vi "GetCurrentXYZPosition (SubVI).vi"(6 ".NET Refnum in - Device":refnum<k24>, 7 "error in (no error)":errorcluster, 10 "Axes Names":string[](array[string])) -> (0 "error out":errorcluster, 1 "Z Position Feedback":dbl, 2 "Y Position Feedback":dbl, 3 "X Position Feedback":dbl, 4 ".NET Refnum out  - Device":refnum<k24>)   [LabVIEW 2016]
uses:
  C:/Users/Aerotech/Documents/BNLStaveAssembly-blueprint/Bin/Aerotech.A3200.dll
  Bin/Aerotech.A3200.dll
panel:
  # "SubVI to retrieve the current position of the XYZ stage"
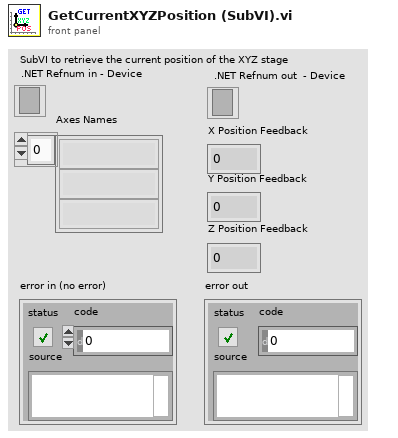
[diagram p1: front panel]
types:
  T1 = cluster{"Axes Names[0]":string, "Axes Names[1]":string, "Axes Names[2]":string, "Axes Names[3]":string, "Axes Names[4]":string, "Axes Names[5]":string, "Axes Names[6]":string, "Axes Names[7]":string, "Axes Names[8]":string}
  T2 = typedef "ControllerDiagPacket.ctl" = cluster{"Number of Diag Packets":i32, "Axes":T3[], "error":errorcluster}
  T3 = typedef "AxisDiagPacket.ctl" = cluster{"Axis Name":string, "Analog Input 0":dbl, "Analog Input 1":dbl, "Axis Fault (num)":i32, "Axis Fault (str)":string, "Axis Fault (bits)":cluster{"AmplifierFault":bool, "AmplifierTemperatureFault":bool, "CcwEndOfTravelLimitFault":bool, "CcwSoftwareLimitFault":bool, "CommunicationLostFault":bool, "CwEndOfTravelLimitFault":bool, "CwSoftwareLimitFault":bool, "EmergencyStopFault":bool, "EncoderFault":bool, "ExternalFault":bool, "FeedbackScalingFault":bool, "GantryMisalignFault ":bool, "HallSensorFault":bool, "InPositionTimeoutFault":bool, "MarkerSearchFault":bool, "MaxVelocityCommandFault":bool, "MissedInterruptFault":bool, "MotorTemperatureFault":bool, "None":bool, "OverCurrentFault":bool, "PositionErrorFault":bool, "PositionFeedbackFault":bool, "PowerSupplyFault":bool, "ProbeInputFault":bool, "SafeZoneFault":bool, "VelocityErrorFault":bool, "VelocityFeedbackFault":bool, "VoltageClampFault":bool}, "Axis Status (num)":i32, "Axis Status (str)":string, "Axis Status (bits)":cluster{"BacklashActive":bool, "CalibrationEnabled1D":bool, "CalibrationEnabled2D":bool, "CommandValid":bool, "DriveAbortPending":bool, "DrivePending":bool, "Enabling":bool, "GainMappingEnabled":bool, "GantryAligned":bool, "GantryRealigning":bool, "Homed":bool, "Homing":bool, "IFOVEnabled":bool, "JogGenerating":bool, "Jogging":bool, "JoystickControl":bool, "MasterSlaveControl":bool, "MotionBlocked":bool, "MotionClamped":bool, "MoveDone":bool, "None":bool, "NotVirtual":bool, "Profiling":bool, "Stability0":bool, "Stability1":bool, "TrajectoryFiltering":bool, "WaitDone":bool}, "Current Command":sgl, "Current Error":sgl, "Current Feedback":sgl, "Digital Inputs":i32, "Digital Outputs":i32, "Drive Status":i32, "Drive Status (str)":string, "Drive Status (bits)":cluster{"AccelerationPhase":bool, "AutofocusActive":bool, "BrakeOutput":bool, "CcwEndOfTravelLimitInput":bool, "CosineEncoderError":bool, "CurrentClamp":bool, "CwEndOfTravelLimitInput":bool, "DecelerationPhase":bool, "DualLoopActive":bool, "EmergencyStopInput":bool, "Enabled":bool, "EncoderClipping":bool, "GalvoCalibrationEnabled":bool, "GalvoPowerCorrection":bool, "HallAInput":bool, "HallBInput":bool, "HallCInput":bool, "HighResolutionMode":bool, "HomeLimitInput":bool, "InPosition":bool, "InPosition2":bool, "MarkerInput":bool, "MarkerLatch":bool, "MoveActive":bool, "NoMotorSupply":bool, "None":bool, "PowerLimiting":bool, "ProgrammingFlash":bool, "ProgrammingMXH":bool, "PSOHaltLatch":bool, "ServoControl":bool, "SineEncoderError":bool}, "Position Feedback Auxiliary":dbl, "Position Command":dbl, "Position Error":dbl, "Position Feedback":dbl, "Program Position Command":dbl, "Program Position Error":dbl, "Program Position Feedback":dbl, "Velocity Command":dbl, "Velocity Error":dbl, "Velocity Feedback":dbl}
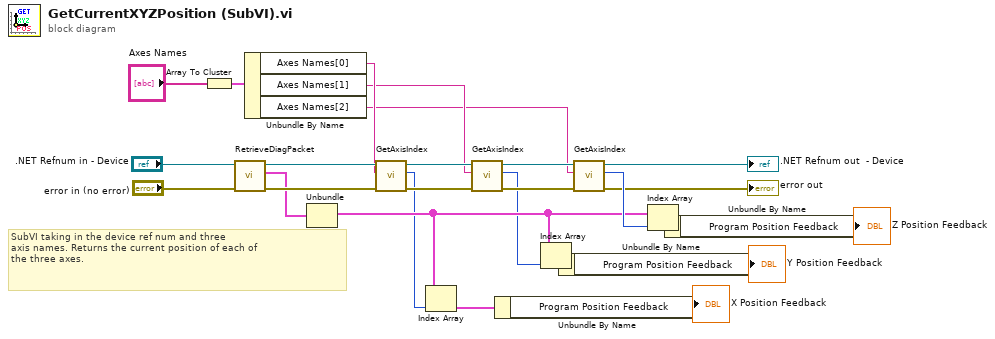
[diagram p0: block diagram]
diagram:
  # "SubVI taking in the device ref num and three\naxis names. Returns the current position of each of\nthe three axes."
  n1 = Array To Cluster(array="Axes Names") -> (cluster=w4:T1)
  n2 = call "RetrieveDiagPacket.vi"("error in (no error)"="error in (no error)", "Controller In"=".NET Refnum in - Device") -> ("error out"=w7:errorcluster, "ControllerDiagPacket"=w6:T2, "Controller Out"=w15:refnum<k24>)  [unwired: 7 in]
  n3 = Unbundle By Name(w4) -> ("Axes Names[0]"=w3:string, "Axes Names[1]"=w2:string, "Axes Names[2]"=w1:string)
  n4 = Unbundle(w6) -> ("Axes"=w21:T3[])  [unwired: 2 out]
  n5 = call "GetAxisIndex.vi"("error in (no error)"=w7, "axis name"=w3, "controller in"=w15) -> ("error out"=w14:errorcluster, "axis index"=w8:i32, "controller out"=w16:refnum<k24>)  [unwired: 6 in]
  n6 = Index Array(array=w21, index=w8) -> (element=w9:T3)
  n7 = call "GetAxisIndex.vi"("error in (no error)"=w14, "axis name"=w2, "controller in"=w16) -> ("error out"=w22:errorcluster, "axis index"=w13:i32, "controller out"=w25:refnum<k24>)  [unwired: 6 in]
  n8 = Unbundle By Name(w9) -> ("Program Position Feedback"=→"X Position Feedback":dbl)
  n9 = Index Array(array=w21, index=w13) -> (element=w12:T3)
  n10 = Unbundle By Name(w12) -> ("Program Position Feedback"=→"Y Position Feedback":dbl)
  n11 = call "GetAxisIndex.vi"("error in (no error)"=w22, "axis name"=w1, "controller in"=w25) -> ("error out"=→"error out":errorcluster, "axis index"=w24:i32, "controller out"=→".NET Refnum out  - Device":refnum<k24>)  [unwired: 6 in]
  n12 = Index Array(array=w21, index=w24) -> (element=w19:T3)
  n13 = Unbundle By Name(w19) -> ("Program Position Feedback"=→"Z Position Feedback":dbl)
